vi "Extract Nom pointe et limite.vi"(0 "Nom pointe de test":string[](array[string]), 2 "Valeur test":string[](array[string]), 3 "Result test":bool[](array[boolean]), 4 "Limit Low":string[](array[string]), 5 "Limit High":string[](array[string])) -> (14 "Nom test":string[](array[string]), 16 "Enfant":cluster{cluster{"élément":string, string}[]}[](array[cluster]), 17 "Result test":bool[](array[boolean]))   [LabVIEW 2020]
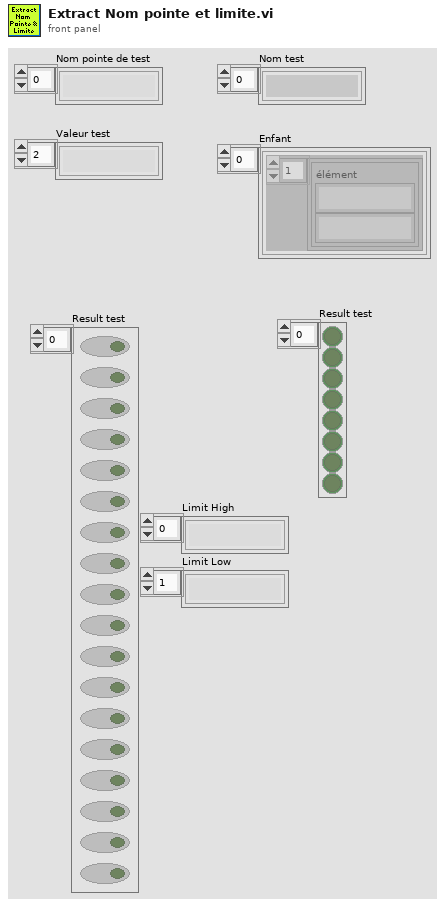
[diagram p1: front panel]
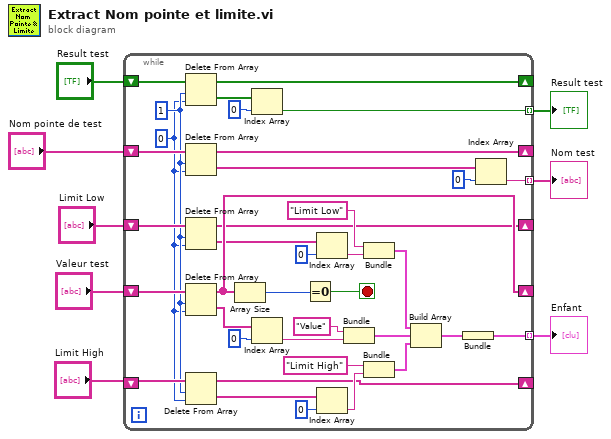
[diagram p0: block diagram]
diagram:
  n1 = while {
    shift-right: [w38] -> _
    shift-left: "Nom pointe de test" -> [w45]
    shift-right: [w41] -> _
    shift-left: "Valeur test" -> [w44]
    tunnel: [w32] -> w6 mode=indexing
    tunnel: [w35] -> w8 mode=indexing
    tunnel: [w29] -> w3 mode=indexing
    shift-right: [w27] -> _
    shift-left: "Result test" -> [w28]
    shift-right: [w10] -> _
    shift-left: "Limit Low" -> [w24]
    shift-right: [w9] -> _
    shift-left: "Limit High" -> [w20]
    stop <- w36 stop-if-true
    w11 = 0 ("indice")
    w19 = 1 ("longueur")
    n2 = Delete From Array(array=w28, length=w19, index=w11) -> (deleted portion=w26:bool[], array with subset deleted=w27:bool[])
    n3 = Delete From Array(array=w45, length=w19, index=w11) -> (deleted portion=w39:string[], array with subset deleted=w38:string[])
    n4 = Delete From Array(array=w24, length=w19, index=w11) -> (deleted portion=w23:string[], array with subset deleted=w10:string[])
    n5 = Delete From Array(array=w44, length=w19, index=w11) -> (deleted portion=w43:string[], array with subset deleted=w41:string[])
    n6 = Delete From Array(array=w20, length=w19, index=w11) -> (deleted portion=w17:string[], array with subset deleted=w9:string[])
    n7 = Array Size(array=w41) -> (size(s)=w37:i32)
    n8 = Index Array(array=w26, index=0 ("indice")) -> (element=w29:bool)
    n9 = Index Array(array=w43, index=0 ("indice")) -> (element=w34:string)
    n10 = Equal To 0?(x=w37) -> (x = 0?=w36:bool)
    n11 = Index Array(array=w23, index=0 ("indice")) -> (element=w14:string)
    n12 = Index Array(array=w17, index=0 ("indice")) -> (element=w16:string)
    n13 = Bundle("élément"="Value", w34) -> (w22:cluster{"élément":string, string})  [unwired: 1 in]
    n14 = Bundle("élément"="Limit Low", w14) -> (w21:cluster{"élément":string, string})  [unwired: 1 in]
    n15 = Bundle("élément"="Limit High", w16) -> (w15:cluster{"élément":string, string})  [unwired: 1 in]
    n16 = Build Array(w21, w22, w15) -> (w33:cluster{"élément":string, string}[])
    n17 = Bundle(w33) -> (w32:cluster{cluster{"élément":string, string}[]})  [unwired: 1 in]
    n18 = Index Array(array=w39, index=0 ("indice")) -> (element=w35:string)
  }
  "Nom test" <- w8
  "Enfant" <- w6
  "Result test" <- w3
